vi "IHL_Stop Collecting.vi"(8 "error in (no error)":errorcluster) -> (0 "error out":errorcluster, 1 "Success":bool, 2 "Array Size":u32, 3 "CD Status":i32)   [LabVIEW 2015, in "Tool Module.lvlib"]
uses:
  Tool Module.lvlib
  _HS Data Stream SM enum--typedef.ctl
  Tool Interface/Tool Interface.lvlib
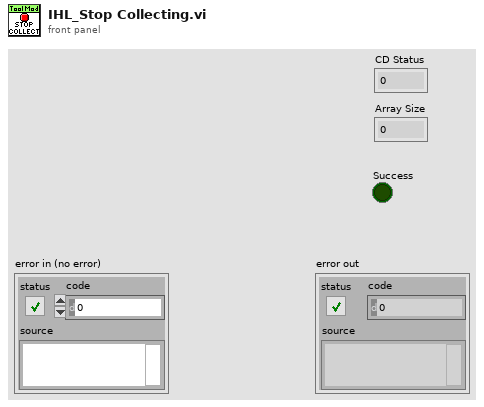
[diagram p1: front panel]
types:
  T1 = typedef "Tool Module.lvlib/_HS Data Stream SM enum--typedef.ctl" = enum16{"Idle", "Receive HS Data", "Close Connection"}
  T2 = typedef "Tool Module.lvlib/_Loop Ctrl Notifiers Cluster--typedef.ctl" = cluster{"Raw Stream Ctrl":refnum<notifier>}
  T3 = typedef "Tool Module.lvlib/_HS Data Stream Params Cluster--typedef.ctl" = cluster{"Raw Data Stream Loop cmd":T1, "Data Array DVR ref":refnum<data-value>, "Sample Data notifier":refnum<notifier>, "Block Count Notifier":refnum<notifier>}
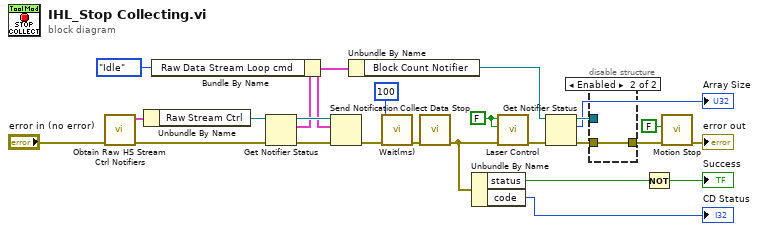
[diagram p0: block diagram]
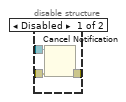
[diagram p2: hidden frame]
diagram:
  w22 = FALSE ("Laser 1")
  n1 = call "Obtain Raw HS Stream Ctrl Notifiers.vi"("error in (no error)"="error in (no error)") -> ("error out"=w17:errorcluster, "Loop Ctrl Notifiers Cluster"=w19:T2)  [unwired: 9 in]
  n2 = Unbundle By Name(w19) -> ("Raw Stream Ctrl"=w18:refnum<notifier>)
  n3 = Get Notifier Status(notifier=w18, error in (no error)=w17) -> (notifier out=w15:refnum<notifier>, current notification=w13:T3, error out=w16:errorcluster)  [unwired: 2 out]
  n4 = Bundle By Name(cluster=w13, "Raw Data Stream Loop cmd"=_HS_Data_Stream_SM_enum--typedef."Idle" ("HS Data Stream SM enum")) -> (w11:T3)
  n5 = Send Notification(notification=w11, notifier=w15, error in (no error)=w16) -> (error out=w24:errorcluster)  [unwired: 1 out]
  n6 = Unbundle By Name(w11) -> ("Block Count Notifier"=w10:refnum<notifier>)
  n7 = call "Wait(ms).vi"("error in (no error)"=w24, "milliseconds"=u32 100) -> ("error out"=w23:errorcluster)  [unwired: 9 in]
  n8 = call "Collect Data Stop.vi"("error in (no error)"=w23) -> ("error out"=w9:errorcluster)  [unwired: 10 in]
  n9 = Unbundle By Name(w9) -> ("status"=w4:bool, "code"=→"CD Status":i32)
  n10 = call "Laser Control.vi"("error in (no error)"=w9, "Laser 2"=w22, "Laser 1"=w22) -> ("error out"=w20:errorcluster)  [unwired: 8 in]
  n11 = Get Notifier Status(notifier=w10, error in (no error)=w20) -> (notifier out=w25:refnum<notifier>, current notification=→"Array Size":u32, error out=w2:errorcluster)  [unwired: 2 out]
  n12 = disable-structure shown="Enabled" {
    disable-tunnel: w25 -> [w28 _]
    disable-tunnel: w2 -> [w27 w29]
    disable-tunnel: [w26 w29] -> w1
    frame Disabled {
      n13 = Cancel Notification(0:w28, 3:w27) -> (11:w26:errorcluster)  [unwired: 2 out]
    }
    frame Enabled {
    }
  }
  n14 = Not(x=w4) -> (.not. x?=→"Success":bool)
  n15 = call "Motion Stop.vi"("error in (no error)"=w1, "Decel?"=FALSE) -> ("error out"=→"error out":errorcluster)  [unwired: 9 in]
